vi "search_radius.vi"(1 "GenAlg_data":T1) -> (0 "Radius":dbl[](array[numeric]))   [LabVIEW 2016]
uses:
  TypeDefs/GenAlg_data.ctl
  TypeDefs/basic_config.ctl
  TypeDefs/element.ctl
  TypeDefs/geration_data.ctl
  TypeDefs/selection_data.ctl
  TypeDefs/SimulatedAnnealing_data.ctl
  TypeDefs/multi_eval_data.ctl
  TypeDefs/termination_data.ctl
panel:
  out "DecayFactor":dbl
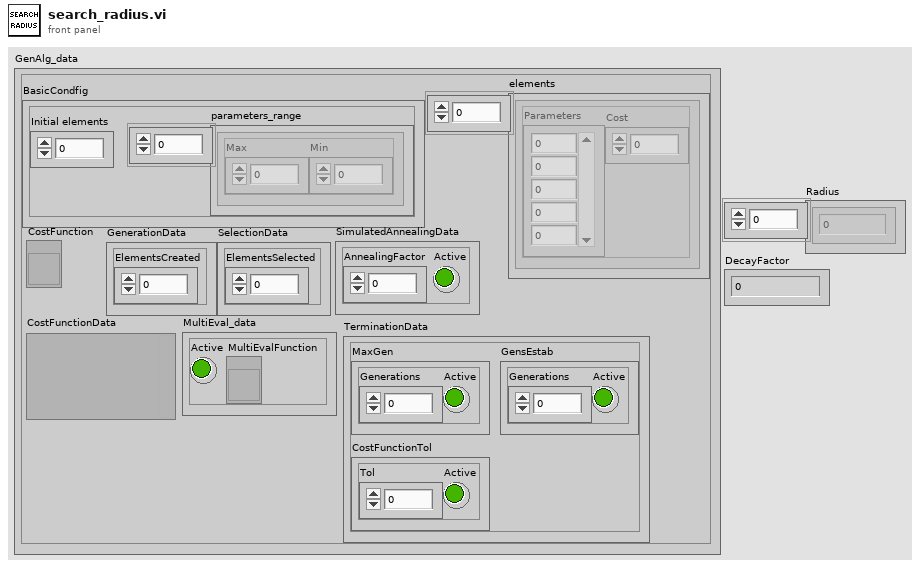
[diagram p1: front panel]
types:
  T1 = typedef "GenAlg_data.ctl" = cluster{"BasicCondfig":T2, "elements":T3[], "CostFunction":refnum<vi>, "GenerationData":T4, "SelectionData":T5, "SimulatedAnnealingData":T6, "CostFunctionData":variant, "MultiEval_data":T7, "TerminationData":T8}
  T2 = typedef "basic_config.ctl" = cluster{"parameters_range":cluster{"Max":dbl, "Min":dbl}[], "Initial elements":i32}
  T3 = typedef "element.ctl" = cluster{"Parameters":dbl[], "Cost":dbl}
  T4 = typedef "geration_data.ctl" = cluster{"ElementsCreated":i32}
  T5 = typedef "selection_data.ctl" = cluster{"ElementsSelected":i32}
  T6 = typedef "SimulatedAnnealing_data.ctl" = cluster{"AnnealingFactor":dbl, "Active":bool}
  T7 = typedef "multi_eval_data.ctl" = cluster{"Active":bool, "MultiEvalFunction":refnum<vi>}
  T8 = typedef "termination_data.ctl" = cluster{"MaxGen":cluster{"Generations":i32, "Active":bool}, "CostFunctionTol":cluster{"Tol":dbl, "Active":bool}, "GensEstab":cluster{"Generations":i32, "Active":bool}}
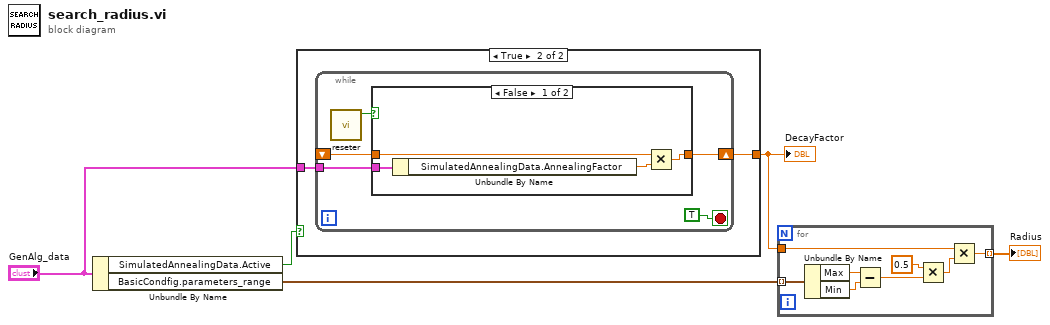
[diagram p0: block diagram]
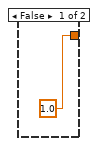
[diagram p2: hidden frame]
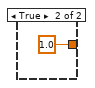
[diagram p3: hidden frame]
diagram:
  n1 = Unbundle By Name("GenAlg_data") -> ("SimulatedAnnealingData.Active"=w3:bool, "BasicCondfig.parameters_range"=w4:cluster{"Max":dbl, "Min":dbl}[])
  n2 = case shown="True" w3 {
    tunnel: "GenAlg_data" -> [_ w8]
    tunnel: [1.0 w7] -> w2
    frame False {
    }
    frame True {
      n3 = while {
        shift-right: [w12] -> w7
        shift-left: _ -> [w10]
        tunnel: w8 -> [w11]
        stop <- TRUE stop-if-true
        n4 = call "reseter.vi"() -> ("Value"=w9:bool)  [unwired: 10 in, 1 out]
        n5 = case shown="False" w9 {
          tunnel: [w14 1.0] -> w12
          tunnel: w11 -> [w17 _]
          tunnel: w10 -> [w15 _]
          frame False {
            n6 = Unbundle By Name(w17) -> ("SimulatedAnnealingData.AnnealingFactor"=w16:dbl)
            n7 = Multiply(x=w15, y=w16) -> (x*y=w14:dbl)
          }
          frame True {
          }
        }
      }
    }
  }
  "DecayFactor" <- w2
  n8 = for {
    tunnel: w4 -> [w26] mode=indexing
    tunnel: w2 -> [w20]
    tunnel: [w19] -> w1 mode=indexing
    n9 = Unbundle By Name(w26) -> ("Max"=w25:dbl, "Min"=w24:dbl)
    n10 = Subtract(x=w25, y=w24) -> (x-y=w23:dbl)
    n11 = Multiply(x=0.5, y=w23) -> (x*y=w21:dbl)
    n12 = Multiply(x=w20, y=w21) -> (x*y=w19:dbl)
  }
  "Radius" <- w1
